vi "EmptyMenu.vi"(8 "error in (no error)":errorcluster, 11 "MenuStrip in":refnum<class "MGI_MenuStrip.lvclass">) -> (0 "error out":errorcluster, 3 "MenuStrip out":refnum<class "MGI_MenuStrip.lvclass">)   [LabVIEW 2016, in "MGI_MenuStrip.lvclass"]
doc: "Removes all menu items from the menu.\n\nAuthored by Derek E. Trepanier\nsupport@mooregoodideas.com\nwww.mooregoodideas.com\n\nCopyright (c) 2012, Moore Good Ideas, Inc.\n\nAll rights reserved.\n\nRedistribution and use in source and binary forms, with or without modification, are permitted provided that the following conditions are met:\n\n * Redistributions of source code must retain the above copyright notice, this list of conditions and the following disclaimer.\n * Redistributions in binary form must reproduce the above copyright notice, this list of conditions and the following disclaimer in the documentation and/or other materials provided with the distribution.\n * Neither the name of Moore Good Ideas, Inc. nor the names of its contributors may be used to endorse or promote products derived from this software without specific prior written permission.\n\nTHIS SOFTWARE IS PROVIDED BY THE COPYRIGHT HOLDERS AND CONTRIBUTORS \"AS IS\" AND ANY EXPRESS OR IMPLIED WARRANTIES, INCLUDING, BUT NOT LIMITED TO, THE IMPLIED WARRANTIES OF MERCHANTABILITY AND FITNESS FOR A PARTICULAR PURPOSE ARE DISCLAIMED. IN NO EVENT SHALL THE COPYRIGHT OWNER OR CONTRIBUTORS BE LIABLE FOR ANY DIRECT, INDIRECT, INCIDENTAL, SPECIAL, EXEMPLARY, OR CONSEQUENTIAL DAMAGES (INCLUDING, BUT NOT LIMITED TO, PROCUREMENT OF SUBSTITUTE GOODS OR SERVICES; LOSS OF USE, DATA, OR PROFITS; OR BUSINESS INTERRUPTION) HOWEVER CAUSED AND ON ANY THEORY OF LIABILITY, WHETHER IN CONTRACT, STRICT LIABILITY, OR TORT (INCLUDING NEGLIGENCE OR OTHERWISE) ARISING IN ANY WAY OUT OF THE USE OF THIS SOFTWARE, EVEN IF ADVISED OF THE POSSIBILITY OF SUCH DAMAGE."
uses:
  <userlib>/_MGI/Menu Building/MenuTypes/MenuStrip/MGI_MenuStrip.lvclass
  <userlib>/_MGI/Menu Building/MenuTypes/MenuStrip/MGI_MenuStrip.lvclass/MGI_MenuStrip.ctl
  System.Windows.Forms
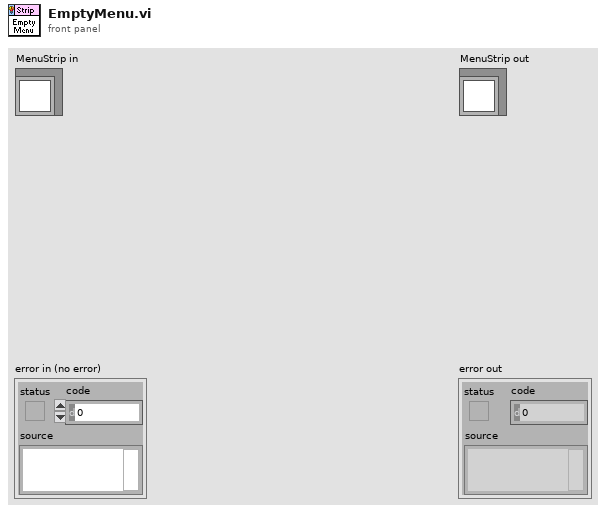
[diagram p1: front panel]
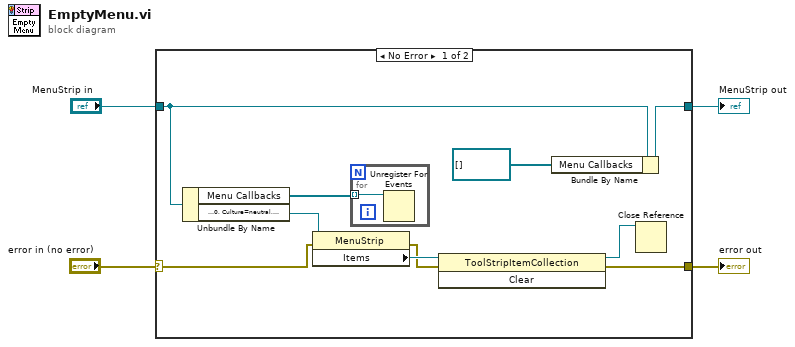
[diagram p0: block diagram]
diagram:
  n1 = case shown="No Error" "error in (no error)" {
    selector: "error in (no error)" -> [w11 w17]
    tunnel: [w9 w17] -> w3
    tunnel: [w6 w16] -> w2
    tunnel: "MenuStrip in" -> [w14 w16]
    frame No Error {
      n2 = Unbundle By Name(w14) -> ("Menu Callbacks"=w7:refnum<k27>[], "MenuStrip"=w13:refnum<k24>)
      n3 = property class="MenuStrip"(reference=w13, error in=w11) -> (error out=w10:errorcluster, "Items"=w12:refnum<k24>)  [unwired: 1 out]
      n4 = for {
        tunnel: w7 -> [w15] mode=indexing
        n5 = Unregister For Events(event registration refnum=w15) -> ()  [unwired: 1 in, 1 out]
      }
      n6 = invoke class="ToolStripItemCollection" method="Clear"(reference=w12, error in=w10) -> (reference out=w8:refnum<k24>, error out=w9:errorcluster)  [unwired: 1 in, 1 out]
      n7 = Bundle By Name(cluster=w14, "Menu Callbacks"=refnum<k27>[] []) -> (w6:refnum<class "MGI_MenuStrip.lvclass">)
      n8 = Close Reference(reference=w8) -> ()  [unwired: 1 in, 1 out]
    }
    frame Error {
    }
  }
  "error out" <- w3
  "MenuStrip out" <- w2
